vi "DIMPowerSupply.ProcPeriodic.vi"(0 "i ref in":refnum<vi>, 3 "ms timeout (10000)":i32=10000, 5 "error in (no error)":errorcluster) -> (14 "i ref out":refnum<vi>, 17 "timed out":bool, 19 "error out":errorcluster)   [LabVIEW 2014, in "DIMPowerSupply.lvlib"]
doc: "This method serves to periodically do things like reading values from the HW. Methods that should be executed periodically should be called from THIS methode. Add code here."
uses:
  DIMPowerSupply.lvlib
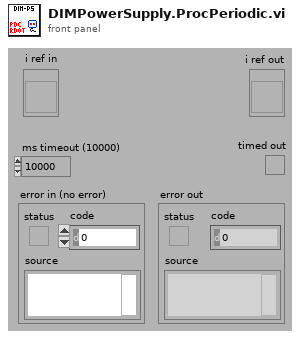
[diagram p1: front panel]
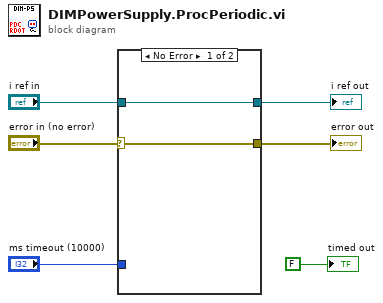
[diagram p0: block diagram]
diagram:
  n1 = case shown="No Error" "error in (no error)" {
    selector: "error in (no error)" -> [w7 w9]
    tunnel: "ms timeout (10000)" -> [_ _]
    tunnel: "i ref in" -> [w8 w10]
    tunnel: [w8 w10] -> w2
    tunnel: [w7 w9] -> w1
    frame No Error {
    }
    frame Error {
    }
  }
  "error out" <- w1
  "i ref out" <- w2
  "timed out" <- FALSE ("timed out")
